vi "Get UDP Settings.vi"(8 "error in (no error)":errorcluster, 11 "Module Configuration":refnum<class "Module Configuration.lvclass">) -> (0 "error out":errorcluster, 2 "UDP configuration":T1={"Device Port Number"=2001, "Device IP"="192.168.1.1.100", "Timeout"=5000, "Port Number"=1234}, 3 "Module Configuration out":refnum<class "Module Configuration.lvclass">)   [LabVIEW 2020, in "Plugin.lvlib" / "Plugin_UI.lvclass"]
doc: "Reads the Hardware Configuration"
uses:
  Plugin_UI.lvclass
  builds/Libraries/LabSys Framework.lvlibp/Configuration Storage/Module Configuration/Module Configuration.lvclass
  UDP Configuration.ctl
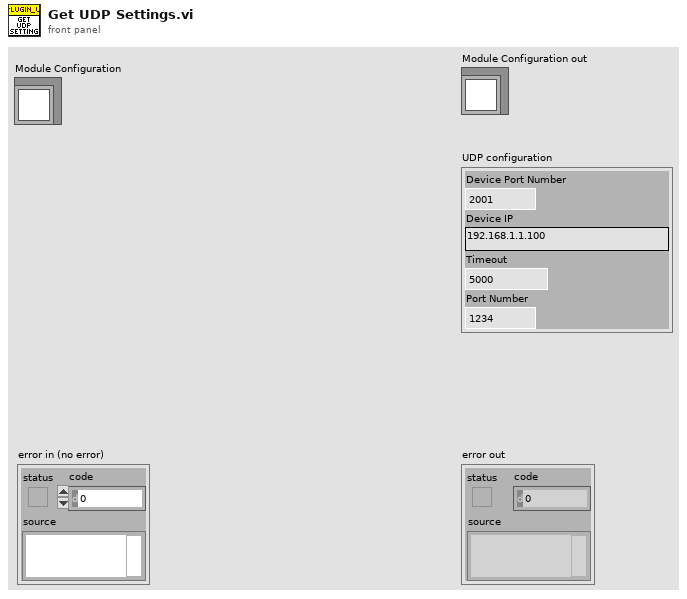
[diagram p1: front panel]
types:
  T1 = typedef "Plugin.lvlib/Plugin_UI.lvclass/UDP Configuration.ctl" = cluster{"Device Port Number":u16, "Device IP":string, "Timeout":i32, "Port Number":u16}
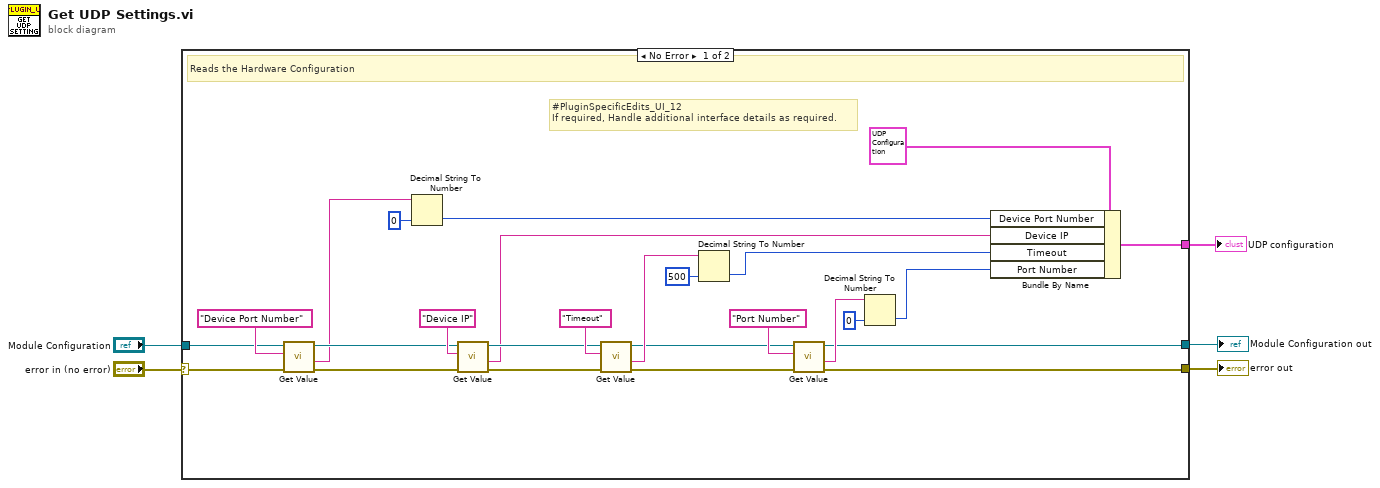
[diagram p0: block diagram]
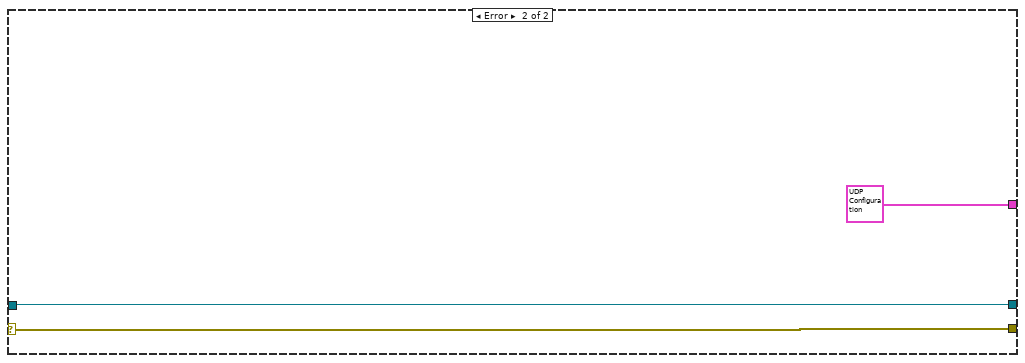
[diagram p2: hidden frame]
diagram:
  n1 = case shown="No Error" "error in (no error)" {
    selector: "error in (no error)" -> [w14 w34]
    tunnel: [w11 w34] -> w4
    tunnel: "Module Configuration" -> [w15 w33]
    tunnel: [w12 w33] -> w2
    tunnel: [w13 T1 {"Device Port Number"=2001, "Device IP"="192.168.1.1.100", "Timeout"=5000, "Port Number"=1234} ("UDP configuration")] -> w1
    frame No Error {
      # "#PluginSpecificEdits_UI_12\nIf required, Handle additional interface details as required."
      # "Reads the Hardware Configuration"
      n2 = call "Get Value.vi"("error in (no error)"=w14, "Key"="Device Port Number", "Module Configuration in"=w15) -> ("error out"=w31:errorcluster, "Value"=w9:string, "Module Configuration out"=w20:refnum<class "Module Configuration.lvclass">)  [unwired: 6 in]
      n3 = Decimal String To Number(string=w9, default (0L)=u16 0 ("default (0 I32)")) -> (number=w8:u16)  [unwired: 1 in, 1 out]
      n4 = call "Get Value.vi"("error in (no error)"=w31, "Key"="Device IP", "Module Configuration in"=w20) -> ("error out"=w30:errorcluster, "Value"=w7:string, "Module Configuration out"=w21:refnum<class "Module Configuration.lvclass">)  [unwired: 6 in]
      n5 = call "Get Value.vi"("error in (no error)"=w30, "Key"="Timeout", "Module Configuration in"=w21) -> ("error out"=w29:errorcluster, "Value"=w27:string, "Module Configuration out"=w22:refnum<class "Module Configuration.lvclass">)  [unwired: 6 in]
      n6 = Decimal String To Number(string=w27, default (0L)=500 ("default (0 I32)")) -> (number=w18:i32)  [unwired: 1 in, 1 out]
      n7 = call "Get Value.vi"("error in (no error)"=w29, "Key"="Port Number", "Module Configuration in"=w22) -> ("error out"=w11:errorcluster, "Value"=w28:string, "Module Configuration out"=w12:refnum<class "Module Configuration.lvclass">)  [unwired: 6 in]
      n8 = Decimal String To Number(string=w28, default (0L)=u16 0 ("default (0 I32)")) -> (number=w19:u16)  [unwired: 1 in, 1 out]
      n9 = Bundle By Name(cluster=T1 {"Device Port Number"=2001, "Device IP"="192.168.1.1.100", "Timeout"=5000, "Port Number"=1234} ("UDP configuration"), "Device Port Number"=w8, "Device IP"=w7, "Timeout"=w18, "Port Number"=w19) -> (w13:T1)
    }
    frame Error {
    }
  }
  "error out" <- w4
  "Module Configuration out" <- w2
  "UDP configuration" <- w1
